vi "Get Result.vi"(8 "error in (no error)":errorcluster, 11 "Channel Scanner Driver in":refnum<class "Channel Scanner Driver.lvclass">) -> (0 "error out":errorcluster, 2 "Result":refnum<class "Acquired Result.lvclass">, 3 "Channel Scanner Driver.lvclass out":refnum<class "Channel Scanner Driver.lvclass">)   [LabVIEW 2019, in "Channel Scanner Driver.lvclass"]
uses:
  Channel Scanner Driver.lvclass
  C:/GitHub/NHMFL_Core/Libraries/Instruments/Instrument Driver/Instrument Driver.lvclass
  Results/Acquired Result/Acquired Result.lvclass
  Channel Scanner Driver.lvclass/Channel Scanner Driver.ctl
  Instrument Driver.lvclass/Instrument Driver.ctl
  Read Scan Channels.vi
  Read Cycle count.vi
  Read Next channel idx.vi
  Read Cycle period.vi
  Simple VISA Reader/Simple VISA Reader Driver.lvclass
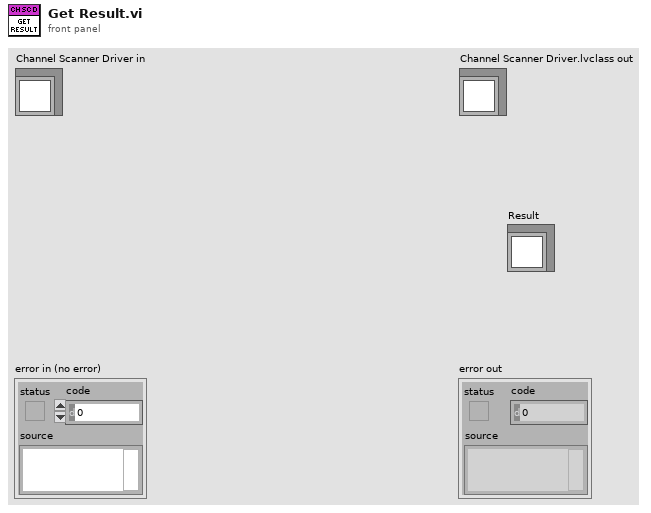
[diagram p1: front panel]
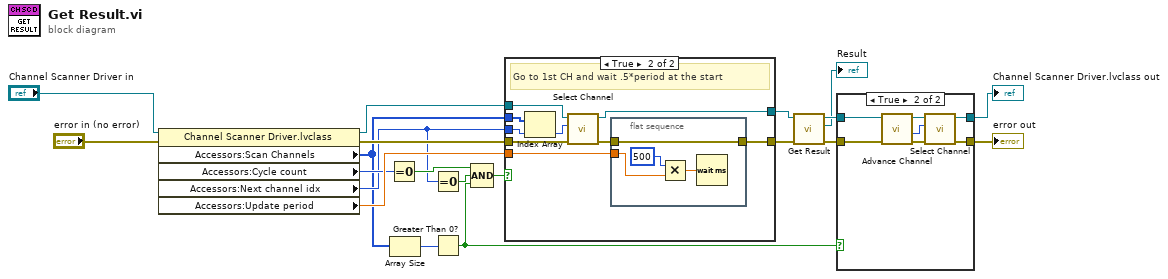
[diagram p0: block diagram]
diagram:
  n1 = property class="Channel Scanner Driver.lvclass"(reference="Channel Scanner Driver in", error in="error in (no error)") -> (reference out=w10:refnum<class "Channel Scanner Driver.lvclass">, error out=w13:errorcluster, "Accessors:Scan Channels"=w2:i32[], "Accessors:Cycle count"=w4:i32, "Accessors:Next channel idx"=w3:i32, "Accessors:Update period"=w12:dbl)
  n2 = Equal To 0?(x=w4) -> (x = 0?=w16:bool)
  n3 = Array Size(array=w2) -> (size(s)=w19:i32)
  n4 = Equal To 0?(x=w3) -> (x = 0?=w14:bool)
  n5 = Greater Than 0?(x=w19) -> (x > 0?=w1:bool)
  n6 = Compound Arithmetic op=AND(w16, w14, w1) -> (w15:bool)
  n7 = case shown="True" w15 {
    tunnel: w13 -> [w22 w24]
    tunnel: w2 -> [_ w31]
    tunnel: w3 -> [_ w30]
    tunnel: [w22 w29] -> w9
    tunnel: w12 -> [_ w28]
    tunnel: w10 -> [w21 w27]
    tunnel: [w21 w23] -> w8
    frame False {
      # "Do nothing"
    }
    frame True {
      # "Go to 1st CH and wait .5*period at the start"
      n8 = Index Array(array=w31, index=w30) -> (element=w26:i32)
      n9 = call-dynamic "Select Channel.vi"("error in (no error)"=w24, "Channel"=w26, "Channel Scanner Driver in"=w27) -> ("error out"=w25:errorcluster, "Channel Scanner Driver out"=w23:refnum<class "Channel Scanner Driver.lvclass">)  [unwired: 7 in]
      n10 = flat-sequence {
        tunnel: w25 -> [w35]
        tunnel: [w35] -> w29
        tunnel: w28 -> [w32]
        frame #0 {
          n11 = Multiply(x=u32 500 ("milliseconds to wait"), y=w32) -> (x*y=w33:dbl)
          n12 = Wait (ms)(milliseconds to wait=w33) -> ()  [unwired: 1 out]
        }
      }
    }
  }
  n13 = call-parent "Get Result.vi"("error in (no error)"=w9, "Simple VISA Reader Driver in"=w8) -> ("error out"=w7:errorcluster, "Result"=→"Result":refnum<class "Acquired Result.lvclass">, "Simple VISA Reader Driver out"=w6:refnum<class "Channel Scanner Driver.lvclass">)  [unwired: 7 in]
  n14 = case shown="True" w1 {
    tunnel: w6 -> [w36 w44]
    tunnel: w7 -> [w37 w43]
    tunnel: [w37 w38] -> w11
    tunnel: [w36 w39] -> w17
    frame False {
    }
    frame True {
      n15 = call-dynamic "Advance Channel.vi"("error in (no error)"=w43, "Channel Scanner Driver in"=w44) -> ("error out"=w41:errorcluster, "Next channel"=w40:i32, "Channel Scanner Driver out"=w42:refnum<class "Channel Scanner Driver.lvclass">)  [unwired: 6 in, 1 out]
      n16 = call-dynamic "Select Channel.vi"("error in (no error)"=w41, "Channel"=w40, "Channel Scanner Driver in"=w42) -> ("error out"=w38:errorcluster, "Channel Scanner Driver out"=w39:refnum<class "Channel Scanner Driver.lvclass">)  [unwired: 7 in]
    }
  }
  "error out" <- w11
  "Channel Scanner Driver.lvclass out" <- w17
